vi "Copy .LLB to NI VeriStand dir.vi"(5 "Files Generated by Build":path[](array[path]), 6 "Top Level/Always Included VIs":path[](array[path]), 7 "Destination Path":path, 8 "error in (no error)":errorcluster, 9 "Target Name":string, 10 "Build Specification Name":string, 11 "Project Path":path) -> (0 "error out":errorcluster)   [LabVIEW 2024]
doc: "This VI is called after each run of a build specification. The VI will copy the generated LLB (Engine or System Explorer) into the VeriStand Custom Device folder (...\\Documents\\National Instruments\\NI VeriStand 2013...)."
uses:
  NationalInstruments.VeriStand
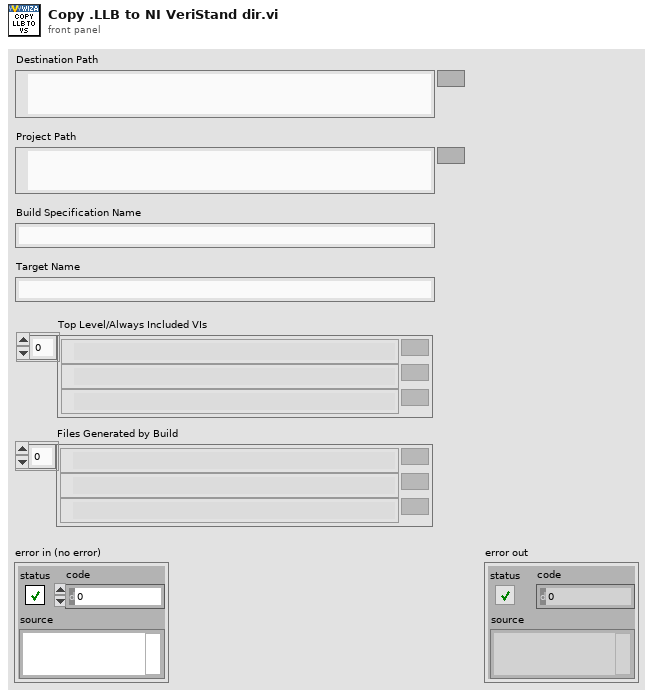
[diagram p1: front panel]
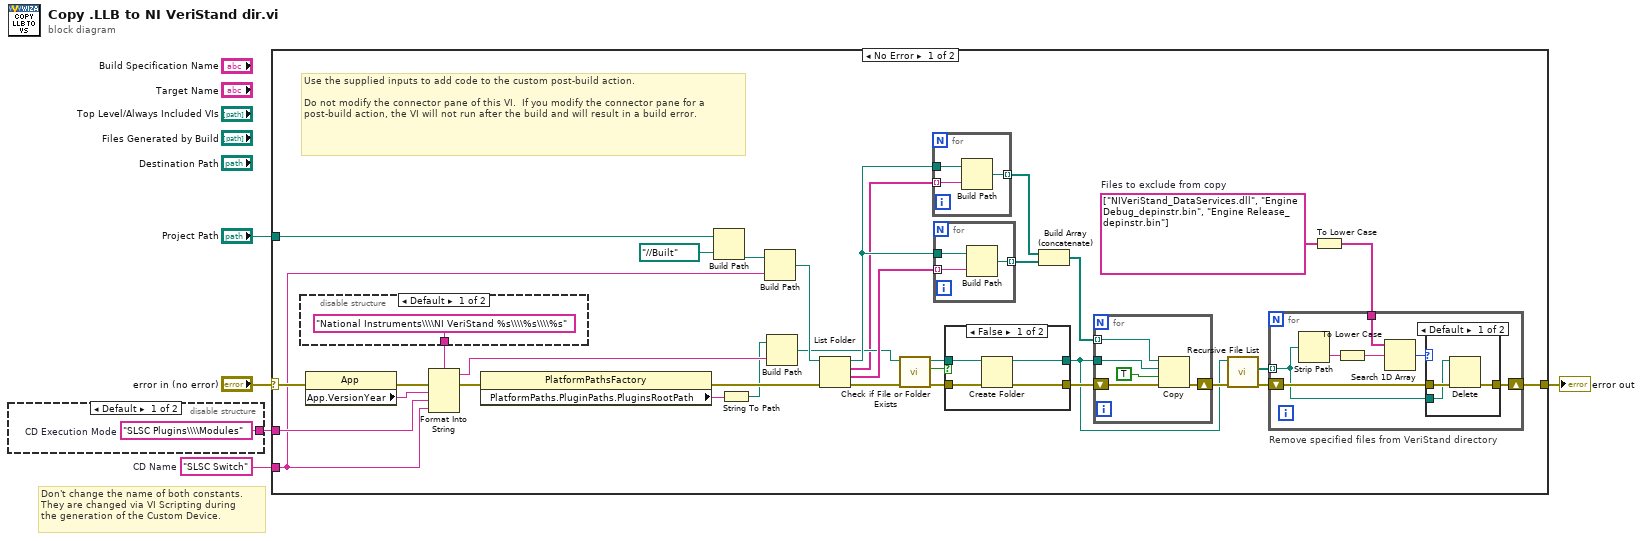
[diagram p0: block diagram]
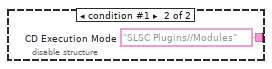
[diagram p2: hidden frame]
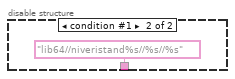
[diagram p3: hidden frame]
diagram:
  w2 = "SLSC Switch"  # CD Name
  # "Don't change the name of both constants.\nThey are changed via VI Scripting during\nthe generation of the Custom Device."
  n1 = disable-structure shown="Default" {
    disable-tunnel: [w6 w7] -> w3
    frame condition #0 (active) {
      w6 = "SLSC Plugins\\\\Modules"  # CD Execution Mode
    }
    frame condition #1 {
      w7 = "SLSC Plugins//Modules"  # CD Execution Mode
    }
  }
  n2 = case shown="No Error" "error in (no error)" {
    selector: "error in (no error)" -> [w25 w72]
    tunnel: [w13 w72] -> w1
    tunnel: "Project Path" -> [w22 _]
    tunnel: w3 -> [w26 _]
    tunnel: w2 -> [w24 _]
    frame No Error {
      w19 = string[] ["NIVeriStand_DataServices.dll", "Engine Debug_depinstr.bin", "Engine Release_depinstr.bin"]  # Files to exclude from copy
      # "Use the supplied inputs to add code to the custom post-build action.\n\nDo not modify the connector pane of this VI.  If you modify the connector pane for a post-build action, the VI will not run after the build and will result in a build error."
      n3 = disable-structure shown="Default" {
        disable-tunnel: ["National Instruments\\\\NI VeriStand %s\\\\%s\\\\%s" ("name or relative path") "lib64//niveristand%s//%s//%s" ("name or relative path")] -> w28
        frame condition #0 (active) {
        }
        frame condition #1 {
        }
      }
      n4 = property class="App"(error in=w25) -> (error out=w30:errorcluster, "App.VersionYear"=w29:string)  [unwired: 1 in, 1 out]
      n5 = Format Into String(format string=w28, error in=w30, w29, w26, w24) -> (resulting string=w31:string, error out=w11:errorcluster)  [unwired: 1 in]
      n6 = property class="PlatformPathsFactory"(error in=w11) -> (error out=w10:errorcluster, "PlatformPaths.PluginPaths.PluginsRootPath"=w9:string)  [unwired: 1 in, 1 out]
      n7 = Build Path(base path=w22, name or relative path=path "../../Built") -> (appended path=w12:path)
      n8 = String To Path(string=w9) -> (path=w8:path)
      n9 = Build Path(base path=w12, name or relative path=w24) -> (appended path=w33:path)
      n10 = Build Path(base path=w8, name or relative path=w31) -> (appended path=w27:path)
      n11 = List Folder(path=w33, error in=w10) -> (path out=w35:path, filenames=w20:string[], folder names=w36:string[], error out=w32:errorcluster)  [unwired: 2 in]
      n12 = call <vilib>:"Check if File or Folder Exists.vi"("error in (no error)"=w32, "path"=w27) -> ("error out"=w37:errorcluster, "file or folder exists?"=w39:bool, "dup path"=w38:path)  [unwired: 7 in]
      n13 = for {
        tunnel: w20 -> [w70] mode=indexing
        tunnel: w35 -> [w71]
        tunnel: [w69] -> w41 mode=indexing
        n14 = Build Path(base path=w71, name or relative path=w70) -> (appended path=w69:path)
      }
      n15 = for {
        tunnel: w36 -> [w67] mode=indexing
        tunnel: w35 -> [w68]
        tunnel: [w66] -> w34 mode=indexing
        n16 = Build Path(base path=w68, name or relative path=w67) -> (appended path=w66:path)
      }
      n17 = case shown="False" w39 {
        tunnel: w38 -> [w58 w60]
        tunnel: w37 -> [w57 w59]
        tunnel: [w56 w60] -> w14
        tunnel: [w55 w59] -> w21
        frame False {
          n18 = Create Folder(path (use dialog)=w58, error in=w57) -> (created path=w56:path, error out=w55:errorcluster)  [unwired: 1 in, 1 out]
        }
        frame True {
        }
      }
      n19 = Build Array (concatenate)(w41, w34) -> (w40:path[])
      n20 = for {
        tunnel: w40 -> [w62] mode=indexing
        shift-right: [w63] -> w15
        shift-left: w21 -> [w64]
        tunnel: w14 -> [w61]
        n21 = Copy(8:w64, 9:TRUE ("overwrite (F)"), 10:w61, 11:w62) -> (0:w63:errorcluster)  [unwired: 1 in, 2 out]
      }
      n22 = call <vilib>:"Recursive File List.vi"("error in (no error)"=w15, "Folder Path"=w14) -> ("error out"=w18:errorcluster, "All Files in Dir"=w17:path[])  [unwired: 5 in, 3 out]
      n23 = To Lower Case(string=w19) -> (all lower case string=w16:string[])
      n24 = for "Remove specified files from VeriStand directory" {
        shift-right: [w45] -> w13
        shift-left: w18 -> [w47]
        tunnel: w17 -> [w44] mode=indexing
        tunnel: w16 -> [w48]
        n25 = Strip Path(path=w44) -> (name=w50:string)  [unwired: 1 out]
        n26 = To Lower Case(string=w50) -> (all lower case string=w49:string)
        n27 = Search 1D Array(1D array=w48, element=w49) -> (index of element=w46:i32)  [unwired: 1 in]
        n28 = case shown="Default" w46 {
          tunnel: w47 -> [w53 w54]
          tunnel: [w52 w54] -> w45
          tunnel: w44 -> [w51 _]
          frame Default {
            n29 = Delete(path (use dialog)=w51, error in=w53) -> (error out=w52:errorcluster)  [unwired: 3 in, 2 out]
          }
          frame -1 {
          }
        }
      }
    }
    frame Error {
    }
  }
  "error out" <- w1
